vi "Waveform Attribute, Filter Labels.vi"(5 "labels":string[](array[string])=["Stim Amp (mA)", "Stim Pulse Width (us)", "Recvy Amp (mA)", "Recvy Pulse Width (us)", "Frequency (Hz)"], 6 "error in":errorcluster, 8 "attributes":T1[](array[typedef])=[{"Label"="Average Size", "Value"=5.0}, {"Label"="Frequency (Hz)", "Value"=21.98167695091432}, {"Label"="NSamp", "Value"=113636.0}, {"Label"="Recvy Amp (mA)", "Value"=0.017683718170655567}, {"Label"="Recvy Amp (mV)", "Value"=176.83718170655567}, {"Label"="Recvy Frequency (Hz)", "Value"=21.981928780026802}, {"Label"="Recvy Pulse Width (us)", "Value"=1521.9629564285276}, {"Label"="Resistance (ohms)", "Value"=10000.0}, {"Label"="Samp Freq (MHz)", "Value"=0.5}, {"Label"="Stim Amp (mA)", "Value"=-0.01711143365109891}, {"Label"="Stim Amp (mV)", "Value"=-171.1143365109891}, {"Label"="Stim Frequency (Hz)", "Value"=21.981425121801834}, {"Label"="Stim Pulse Width (us)", "Value"=1505.3487195968626}, {"Label"="dt (us)", "Value"=2.0}] {"Value" format="%#.3f"}) -> (0 "error out":errorcluster, 2 "filtered results":T1[](array[typedef]) {"Value" format="%#.3f"})   [LabVIEW 2010]
doc: "This function acts as a bandpass filter for the selected waveform attributes."
uses:
  Waveform Attribute Cluster.ctl
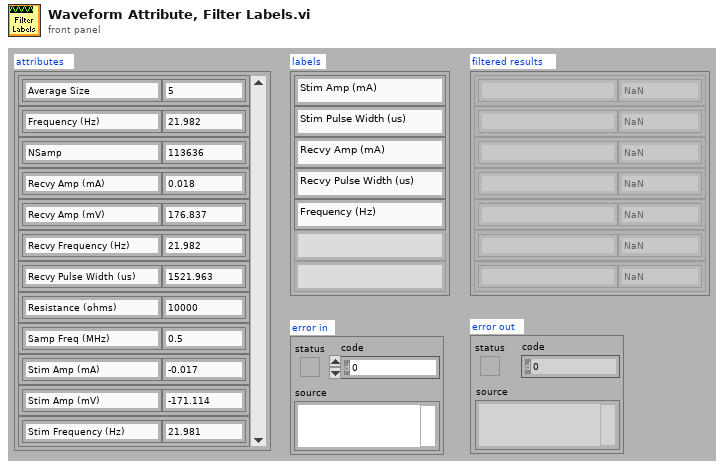
[diagram p1: front panel]
types:
  T1 = typedef "Waveform Attribute Cluster.ctl" = cluster{"Label":string, "Value":dbl}
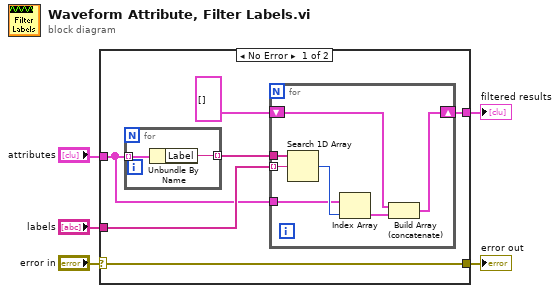
[diagram p0: block diagram]
diagram:
  n1 = case shown="No Error" "error in" {
    selector: "error in" -> [w6 w21]
    tunnel: "labels" -> [w10 _]
    tunnel: "attributes" -> [w9 _]
    tunnel: [w8 _] -> w3
    tunnel: [w6 w21] -> w1
    frame No Error {
      n2 = for {
        tunnel: w9 -> [w20] mode=indexing
        tunnel: [w19] -> w11 mode=indexing
        n3 = Unbundle By Name(w20) -> ("Label"=w19:string)
      }
      n4 = for {
        tunnel: w11 -> [w18]
        tunnel: w10 -> [w17] mode=indexing
        shift-right: [w12] -> w8
        shift-left: cluster{"Label":string, "Value":dbl}[] [] -> [w13]
        tunnel: w9 -> [w15]
        n5 = Search 1D Array(1D array=w18, element=w17) -> (index of element=w16:i32)  [unwired: 1 in]
        n6 = Index Array(array=w15, index=w16) -> (element=w14:T1)
        n7 = Build Array (concatenate)(w13, w14) -> (w12:T1[])
      }
    }
    frame Error {
    }
  }
  "filtered results" <- w3
  "error out" <- w1
